vi "ITX to LV 2.2.vi"(0 "file (use dialog)":path=path "P:/sample/GaAs/GaAs quantum dots/2008/PL Map/A1 735/060731ASBA_A1_6.0.itx") -> (2 "2D array":dbl[][](array[numeric]), 3 "1D arrays":dbl[][](array[numeric]), 4 "wave names":string[](array[string]), 5 "Notes":string)   [LabVIEW 2016, in "LV to ITX.lvclass"]
uses:
  LV to ITX.lvclass
panel:
  out "variant to data (ms)":u32
  out "Commands":string
  out "parse 2 (ms)":u32
  out "text to data (ms)":u32
  out "parse 1 (ms)":u32
  out "open file (ms)":u32
  out "Array 4":i32[](array[numeric])
  out "Array":string[](array[string])
  out "array":string[](array[string])
  out "error out":errorcluster
  out "logical AND":bool
  out "Array 2":string[](array[string])
  out "spreadsheet strings":string[](array[string])
  in  "error in":errorcluster
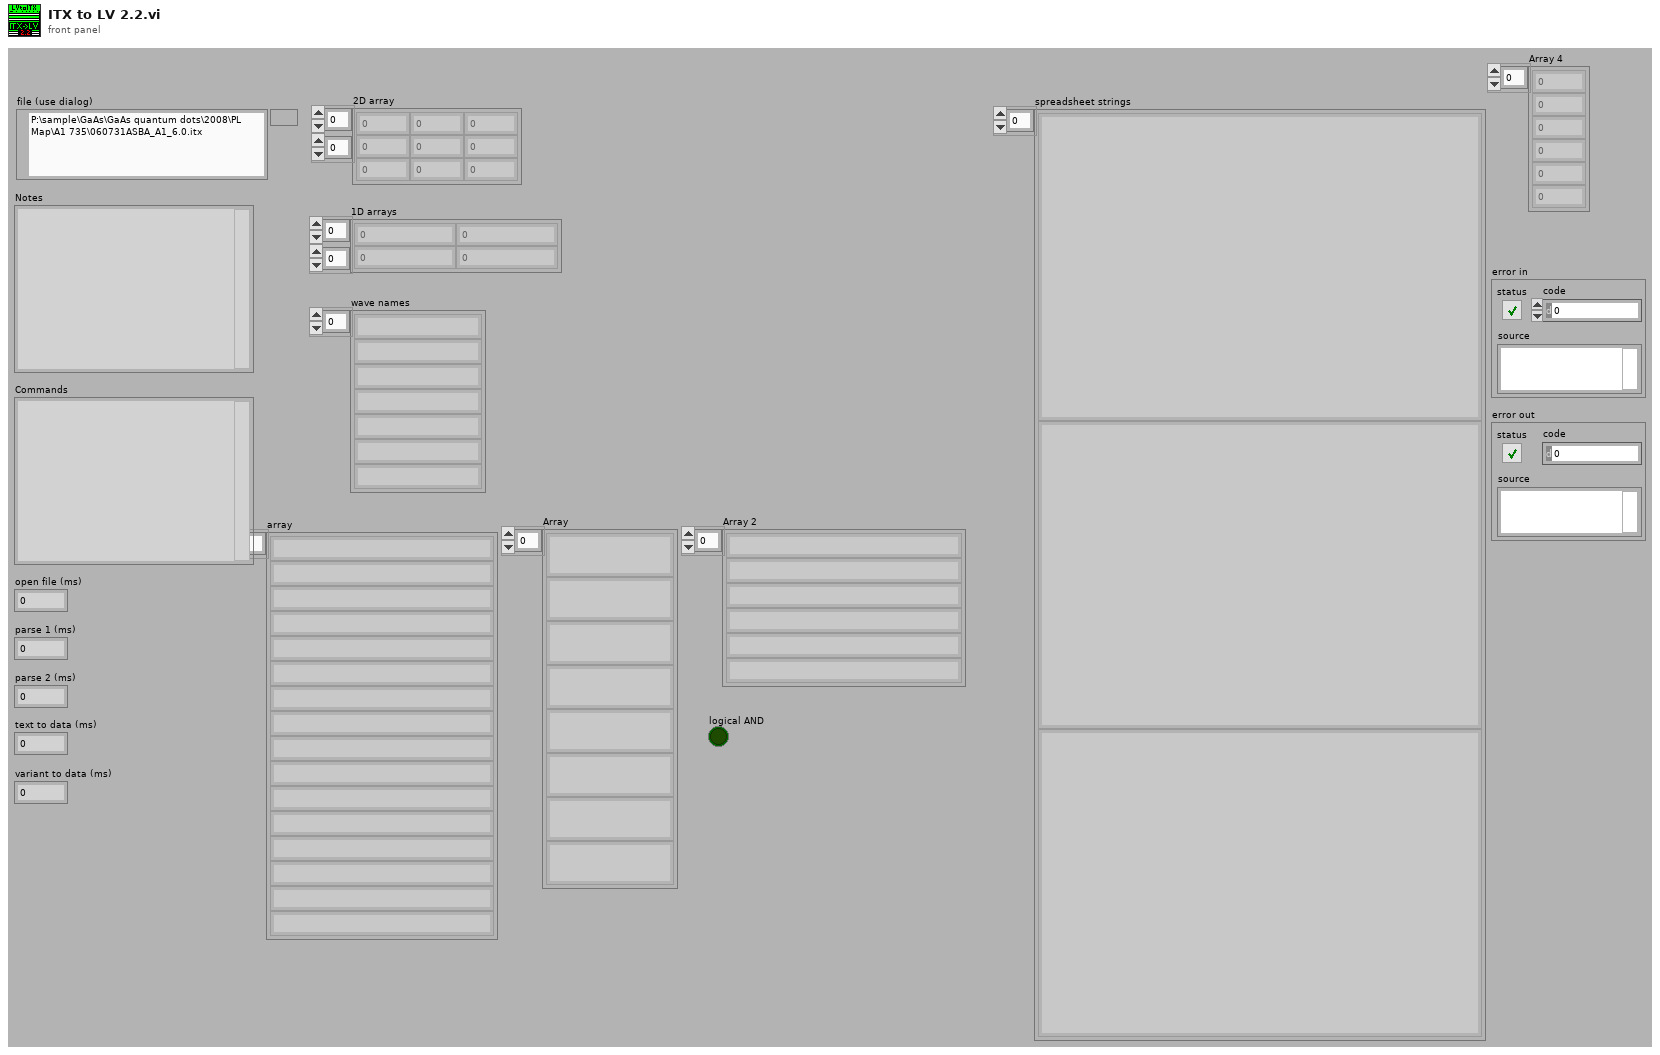
[diagram p1: front panel]
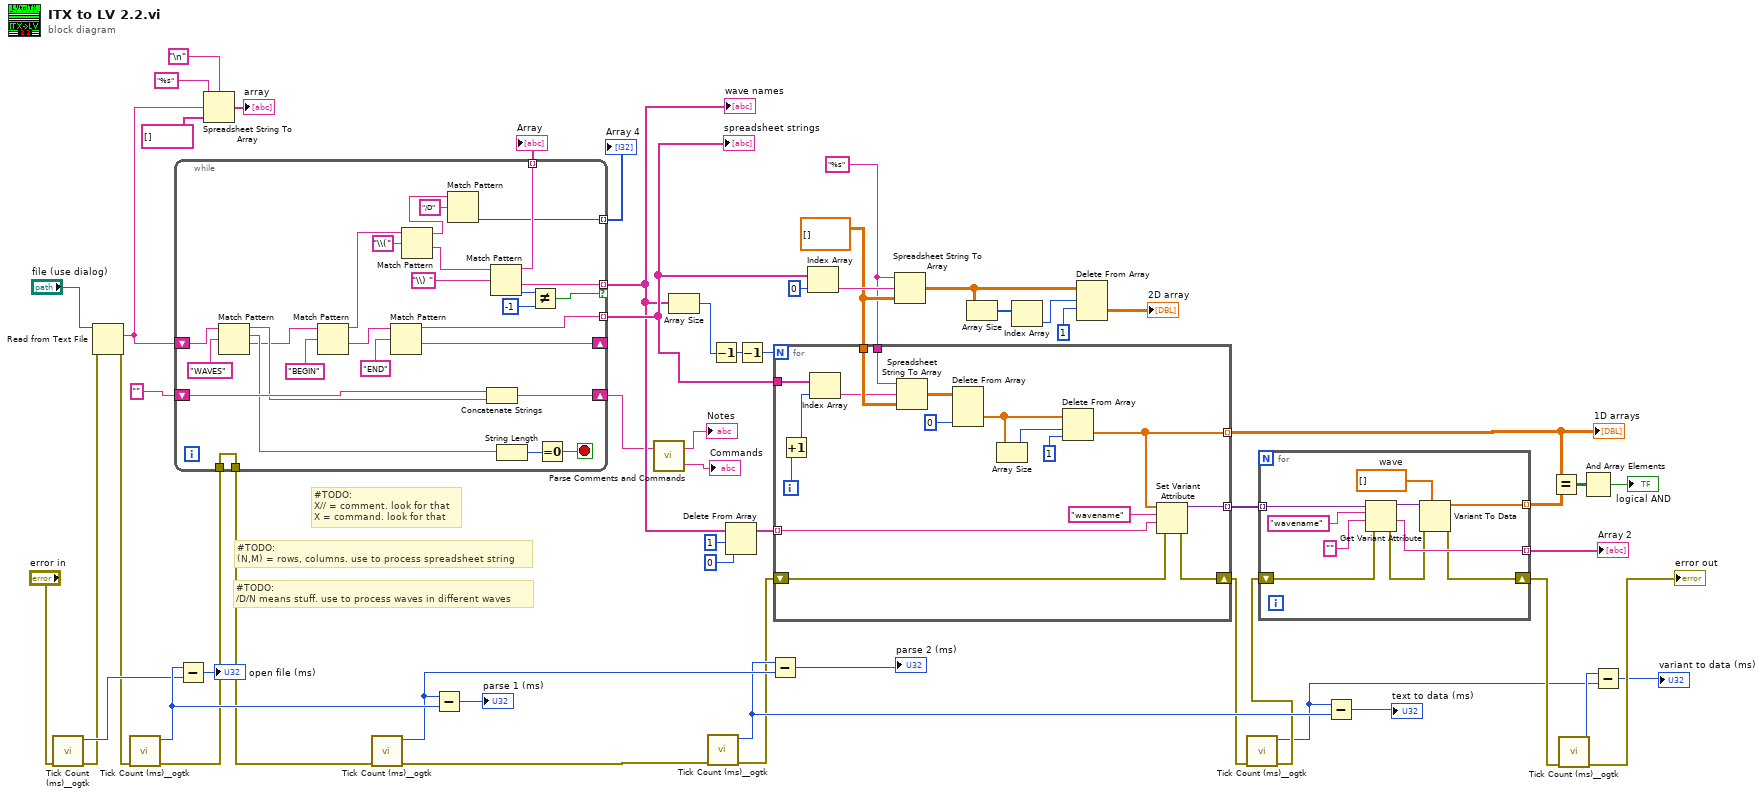
[diagram p0: block diagram]
diagram:
  w49 = "%s" ("format string")
  w50 = dbl[][] [] ("array type (2D Dbl)")
  # "#TODO:\n/D/N means stuff. use to process waves in different waves"
  # "#TODO:\n(N,M) = rows, columns. use to process spreadsheet string"
  # "#TODO:\nX// = comment. look for that\nX = command. look for that"
  n1 = call <userlib>:"Tick Count (ms)__ogtk.vi"("error in (no error)"="error in") -> ("error out"=w16:errorcluster, "millisecond timer value"=w19:u32)  [unwired: 9 in]
  n2 = Read from Text File(file (use dialog)="file (use dialog)", error in=w16) -> (text=w29:string, error out=w10:errorcluster)  [unwired: 1 in, 3 out]
  n3 = call <userlib>:"Tick Count (ms)__ogtk.vi"("error in (no error)"=w10) -> ("error out"=w15:errorcluster, "millisecond timer value"=w23:u32)  [unwired: 9 in]
  n4 = while {
    tunnel: [w63] -> w34 mode=indexing
    shift-right: [w83] -> _
    shift-left: w29 -> [w75]
    tunnel: [w67] -> w33 mode=indexing if=w59
    shift-right: [w77] -> w13
    shift-left: "" ("regular expression") -> [w76]
    tunnel: [w69] -> w27 mode=indexing
    tunnel: [w64] -> w26 mode=indexing
    tunnel: w15 -> [w58]
    tunnel: [w58] -> w14
    stop <- w62 stop-if-true
    n5 = Match Pattern(string=w75, regular expression="WAVES") -> (before substring=w73:string, match substring=w74:string, after substring=w72:string)  [unwired: 2 out]
    n6 = Match Pattern(string=w72, regular expression="BEGIN" ("regular expression 2")) -> (before substring=w70:string, after substring=w84:string)  [unwired: 3 out]
    n7 = Match Pattern(string=w84, regular expression="END" ("regular expression 3")) -> (before substring=w63:string, after substring=w83:string)  [unwired: 3 out]
    n8 = Match Pattern(string=w70, regular expression="\\(") -> (before substring=w65:string, after substring=w68:string)  [unwired: 3 out]
    n9 = Match Pattern(string=w65, regular expression="/D") -> (offset past match=w64:i32)  [unwired: 4 out]
    n10 = Concatenate Strings(w76, w73) -> (w77:string)
    n11 = Match Pattern(string=w68, regular expression="\\) ") -> (before substring=w69:string, after substring=w67:string, offset past match=w61:i32)  [unwired: 2 out]
    n12 = String Length(string=w74) -> (length=w82:i32)
    n13 = Not Equal?(x=w61, y=-1) -> (x != y?=w59:bool)
    n14 = Equal To 0?(x=w82) -> (x = 0?=w62:bool)
  }
  "wave names" <- w33
  "spreadsheet strings" <- w34
  "Array" <- w27
  "Array 4" <- w26
  n15 = Subtract(x=w23, y=w19) -> (x-y=→"open file (ms)":u32)
  n16 = Spreadsheet String To Array(delimiter (Tab)="\n", format string="%s", spreadsheet string=w29, array type (2D Dbl)=string[] []) -> (array=→"array":string[])
  n17 = call <userlib>:"Tick Count (ms)__ogtk.vi"("error in (no error)"=w14) -> ("error out"=w1:errorcluster, "millisecond timer value"=w21:u32)  [unwired: 9 in]
  n18 = Subtract(x=w21, y=w23) -> (x-y=→"parse 1 (ms)":u32)
  n19 = call "Parse Comments and Commands.vi"("ITX Notes and Commands"=w13) -> ("Commands"=→"Commands":string, "Notes"=→"Notes":string)  [unwired: 1 in]
  n20 = Array Size(array=w33) -> (size(s)=w35:i32)
  n21 = call <userlib>:"Tick Count (ms)__ogtk.vi"("error in (no error)"=w1) -> ("error out"=w9:errorcluster, "millisecond timer value"=w18:u32)  [unwired: 9 in]
  n22 = Decrement(x=w35) -> (x-1=w48:i32)
  n23 = Delete From Array(array=w33, length=1, index=0) -> (array with subset deleted=w43:string[])  [unwired: 1 out]
  n24 = Decrement(x=w48) -> (x-1=w47:i32)
  n25 = Subtract(x=w18, y=w21) -> (x-y=→"parse 2 (ms)":u32)
  n26 = for {
    N: w47 -> [_]
    tunnel: [w85] -> w38 mode=indexing
    tunnel: w50 -> [w96]
    tunnel: w34 -> [w95]
    tunnel: w49 -> [w94]
    tunnel: w43 -> [w89] mode=indexing
    tunnel: [w88] -> w40 mode=indexing
    shift-right: [w87] -> w8
    shift-left: w9 -> [w86]
    i -> [w93]
    n27 = Increment(x=w93) -> (x+1=w92:i32)
    n28 = Index Array(array=w95, index=w92) -> (element=w91:string)
    n29 = Spreadsheet String To Array(format string=w94, spreadsheet string=w91, array type (2D Dbl)=w96) -> (array=w100:dbl[][])  [unwired: 1 out]
    n30 = Delete From Array(array=w100, index (col)=0 ("disabled index (col)")) -> (deleted portion=w99:dbl[])  [unwired: 2 in, 1 out]
    n31 = Array Size(array=w99) -> (size(s)=w98:i32)
    n32 = Delete From Array(array=w99, length=w98, index=1) -> (deleted portion=w85:dbl[])  [unwired: 1 out]
    n33 = Set Variant Attribute(Variant=w85, name="wavename", value=w89, error in=w86) -> (Variant out=w88:variant, error out=w87:errorcluster)  [unwired: 1 out]
  }
  "1D arrays" <- w38
  n34 = Index Array(array=w34, index=0) -> (element=w56:string)
  n35 = Spreadsheet String To Array(format string=w49, spreadsheet string=w56, array type (2D Dbl)=w50) -> (array=w54:dbl[][])  [unwired: 1 out]
  n36 = Array Size(array=w54) -> (size(s)=w53:i32[])
  n37 = Index Array(array=w53) -> (element=w51:i32)  [unwired: 1 in]
  n38 = Delete From Array(array=w54, length=w51, index (row)=1) -> (deleted portion=→"2D array":dbl[][])  [unwired: 1 in, 1 out]
  n39 = call <userlib>:"Tick Count (ms)__ogtk.vi"("error in (no error)"=w8) -> ("error out"=w7:errorcluster, "millisecond timer value"=w2:u32)  [unwired: 9 in]
  n40 = for {
    tunnel: [w108] -> w41 mode=indexing
    tunnel: w40 -> [w109] mode=indexing
    shift-right: [w103] -> w6
    shift-left: w7 -> [w102]
    tunnel: [w104] -> w39 mode=indexing
    w105 = dbl[] []  # wave
    n41 = Get Variant Attribute(Variant=w109, name="wavename", default value (empty Variant)="" ("name"), error in=w102) -> (duplicate Variant=w106:variant, value=w108:string, error out=w107:errorcluster)  [unwired: 1 out]
    n42 = Variant To Data(error in=w107, type=w105, Variant=w106) -> (data=w104:dbl[], error out=w103:errorcluster)
  }
  "Array 2" <- w41
  n43 = Subtract(x=w2, y=w18) -> (x-y=→"text to data (ms)":u32)
  n44 = Equal?(x=w38, y=w39) -> (x = y?=w37:bool[][])
  n45 = call <userlib>:"Tick Count (ms)__ogtk.vi"("error in (no error)"=w6) -> ("error out"=→"error out":errorcluster, "millisecond timer value"=w3:u32)  [unwired: 9 in]
  n46 = And Array Elements(Boolean array=w37) -> (logical AND=→"logical AND":bool)
  n47 = Subtract(x=w3, y=w2) -> (x-y=→"variant to data (ms)":u32)
